vi "Actor Core.vi"(8 "error in":errorcluster, 11 "BooleanView In":refnum<class "BooleanView.lvclass">) -> (0 "error out":errorcluster, 3 "Actor out":refnum<class "Actor.lvclass">)   [LabVIEW 2017, in "MVA Example.lvlib" / "BooleanView.lvclass"]
doc: "(<B>Filename</B>: Actor Framework.lvlib:Actor.lvclass:Actor Core.vi)\n\nReceives messages to the actor, reacts to them, and initiates any error handling that may shut the actor down.\n\nDescendant classes may override this VI to append parallel tasks for the actor to complete while it handles messages. Overrides use the Call Parent Method node.\n\n<License>\nCopyright © 2017 Composed Systems, LLC | All rights reserved\nwww.composed.io\n\nAuthor: Ethan Stern <ethan.stern@composed.io>\n\nThis software is provided \"AS IS\" WITHOUT WARRANTIES, either express or implied, AND IS FOR EDUCATIONAL PURPOSES ONLY.\n</License>MVA Framework 1.6.0.31\nEthan Stern - Composed Systems\nCopyright (c) 2018, Composed Systems"
uses:
  BooleanView.lvclass
  <vilib>/ActorFramework/Actor/Actor.lvclass
  <vilib>/Composed Systems/MVA Framework/Framework/IViewable/IViewable/IViewable.lvclass
panel:
  out "Boolean 3":bool
  out "Boolean 2":bool
  out "Boolean 1":bool
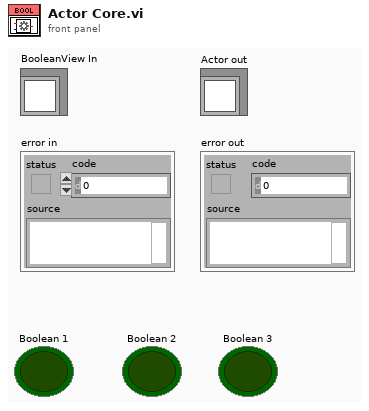
[diagram p1: front panel]
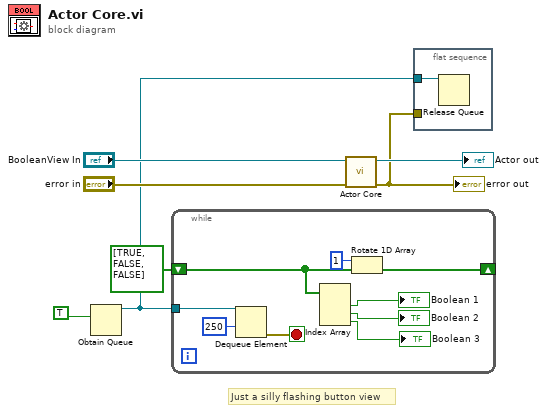
[diagram p0: block diagram]
diagram:
  # "Just a silly flashing button view"
  n1 = Obtain Queue(element data type=TRUE) -> (queue out=w3:refnum<queue>)  [unwired: 4 in, 2 out]
  n2 = while {
    tunnel: w3 -> [w16]
    shift-right: [w13] -> _
    shift-left: bool[] [TRUE, FALSE, FALSE] -> [w11]
    stop <- w14 stop-if-true
    n3 = Dequeue Element(queue=w16, timeout in ms (-1)=250) -> (error out=w14:errorcluster)  [unwired: 1 in, 3 out]
    n4 = Index Array(array=w11) -> (element #1=→"Boolean 1":bool, element #2=→"Boolean 2":bool, element #3=→"Boolean 3":bool)  [unwired: 3 in]
    n5 = Rotate 1D Array(1:w11, 2:1 ("n")) -> (0:w13:bool[])
  }
  n6 = call-parent "Actor Core.vi"("error in"="error in", "IViewable In"="BooleanView In") -> ("error out"=w1:errorcluster, "Actor out"=→"Actor out":refnum<class "Actor.lvclass">)  [unwired: 8 in]
  "error out" <- w1
  n7 = flat-sequence {
    tunnel: w3 -> [w17]
    tunnel: w1 -> [_]
    frame #0 {
      n8 = Release Queue(queue=w17) -> ()  [unwired: 2 in, 3 out]
    }
  }
